vi "External EEPROM.vi"(8 "error in":errorcluster) -> (0 "error out":errorcluster, 2 "Pass?":bool, 3 "VISA resource name out":refnum<visa-resource-name>)   [LabVIEW 2009]
uses:
  Digit IO PCI 6503/Digit IO control.ctl
  Global/Global 1.vi
  <vilib>/Instr/_visa.llb/VISA Configure Serial Port (Instr).vi
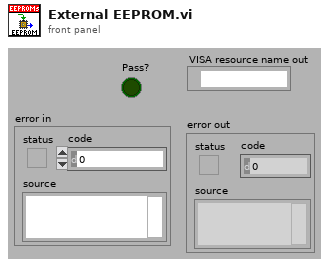
[diagram p1: front panel]
types:
  T1 = typedef "Digit IO control.ctl" = enum16{"Pull X1_4 Low", "Disconnect Pull X1_4 Low", "Down Cylinder", "Disconnect Down Cylinder", "Load X1_1_5", "Disconnect Load X1_1_5", "Measu X1_1_5", "Disconnect Measu X1_1_5", "Measu Z1_1_5", "Disconnect Measu Z1_1_5", "Power X1_1", "Disconnect Power X1_1", "RS232 Power", "Disconnect RS232 Power", "Card Cylinder", "Disconnect Card Cylinder", "Fail LED", "Disconnect Fail LED", "LCA Power", "Disconnect LCA Power", "BeyondCylinderDowndigit", "Disconnect BeyondCylinderDowendigit", "Frequency", "Disconnect Frequency", "Measu Current", "Disconnect Measu Current", "Measu current_1", "Disconnect Measu current_1", "Digit ALL", "Disconnect Digit ALL", "PASS LED", "Disconnect PASS LED", "Load Z1_1_3", "Disconnect Load Z1_1_3", "RS232 Connect", "Disconnect RS232 Connect", "Power Z1_7", "Disconnect Power Z1_7", "Pull Z_1_5  low", "Disconnect Pull Z_1_5  low", "Connect LCA_1", "Disconnect LCA_1", "short LCA", "Disconnect short LCA", "PT100", "Disconnect PT100", "NO connect", "Disconnect NO connect"}
  T2 = cluster{"People":string, "product  number":string, "Test time":string, "VHeatFuse_noload":string, "VHeatFuse_load":string, "VoverrideDiode":string, "Test firmware upload via X1":string, "TemperAddress":string, "Troom":string, "TLCU":string, "Adjustment factor":string, "MeasuredFreq":string, "I2C communication":string, "Light-emitting diode on Z2":string, "Battery warning/inhibit":string, "Reset by IC10":string, "External EEPROM":string, "RFID card detection and reading RFID":string, "Production parameters in internal EEPROM":string, "Current consumption in sleep mode":string, "Application and database upload":string, "Test result":string, "Table head[22]":string, "Table head[23]":string}
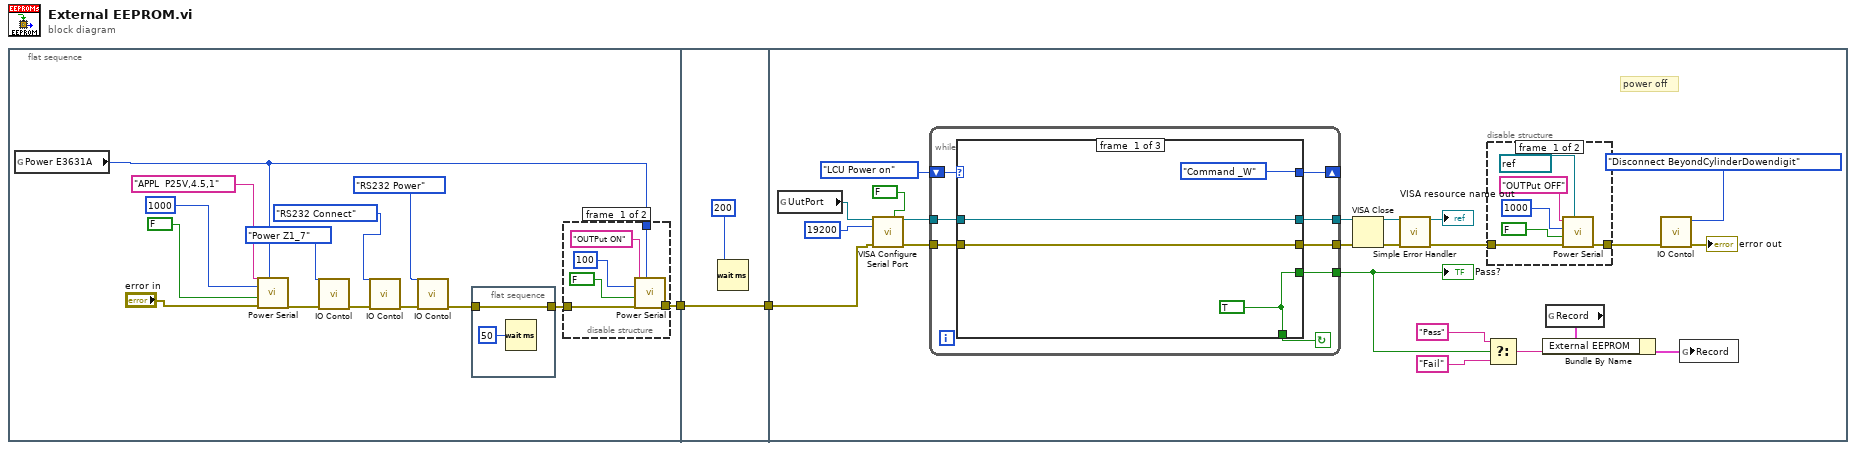
[diagram p0: block diagram]
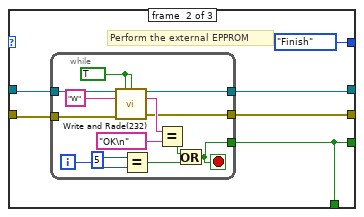
[diagram p4: hidden frame]
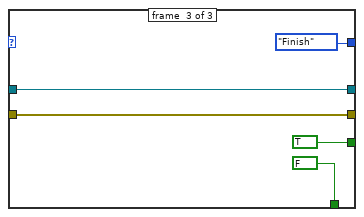
[diagram p5: hidden frame]
diagram:
  n1 = flat-sequence {
    tunnel: [w4] -> w1
    tunnel: [w26] -> w2
    tunnel: w1 -> [w26]
    tunnel: w2 -> [w35]
    frame #0 {
      n2 = global read "Global 1.vi" "Power E3631A"() -> (w7:i32)
      n3 = call "Power Serial.vi"("VISA Resource Address"=w7, "error in (no error)"="error in", "Rd?"=FALSE, "Delay"=1000, "IN"="APPL  P25V,4.5,1" ("In")) -> ("error out"=w11:errorcluster)  [unwired: 6 out]
      n4 = call "IO Contol.vi"("error in"=w11, "IO Operation"=Digit_IO_control."Power Z1_7" ("Enum")) -> ("error out"=w12:errorcluster)  [unwired: 9 out]
      n5 = call "IO Contol.vi"("error in"=w12, "IO Operation"=Digit_IO_control."RS232 Connect" ("Enum")) -> ("error out"=w13:errorcluster)  [unwired: 9 out]
      n6 = call "IO Contol.vi"("error in"=w13, "IO Operation"=Digit_IO_control."RS232 Power" ("Enum")) -> ("error out"=w6:errorcluster)  [unwired: 9 out]
      n7 = flat-sequence {
        tunnel: [w25] -> w5
        tunnel: w6 -> [w25]
        frame #0 {
          n8 = Wait (ms)(milliseconds to wait=u32 50) -> ()  [unwired: 1 out]
        }
      }
      n9 = disable-structure shown="Enabled" {
        disable-tunnel: w7 -> [w19 _]
        disable-tunnel: w5 -> [w18 w23]
        disable-tunnel: [w17 w23] -> w4
        frame #0 {
          n10 = call "Power Serial.vi"("VISA Resource Address"=w19, "error in (no error)"=w18, "Rd?"=FALSE, "Delay"=100, "IN"="OUTPut ON" ("In")) -> ("error out"=w17:errorcluster)  [unwired: 5 in, 1 out]
        }
        frame #1 {
        }
      }
    }
    frame #1 {
      n11 = Wait (ms)(milliseconds to wait=u32 200) -> ()  [unwired: 1 out]
    }
    frame #2 {
      # "power off"
      n12 = global read "Global 1.vi" "UutPort"() -> (w34:refnum<visa-resource-name>)
      n13 = call-poly "VISA Configure Serial Port"("VISA resource name"=w34, "Enable Termination\nChar (T)"=FALSE ("Enable Termination\nChar (T)"), "baud rate (9600)"=u32 19200, "error in (no error)"=w35) -> ("VISA resource name out"=w38:refnum<visa-resource-name>, "error out"=w36:errorcluster)  [unwired: 3 in, 7 out]
      n14 = while {
        shift-right: [w55] -> _
        shift-left: enum16{"LCU Power on", "Command _W", "Finish"}."LCU Power on" -> [w56]
        tunnel: [w61] -> w39
        tunnel: w38 -> [w60]
        tunnel: [w59] -> w37
        tunnel: w36 -> [w58]
        tunnel: [w57] -> w30
        stop <- w62 continue-if-true
        n15 = case shown="\"Command _W\"" w56 {
          tunnel: [enum16{"LCU Power on", "Command _W", "Finish"}."Command _W" enum16{"LCU Power on", "Command _W", "Finish"}."Finish" enum16{"LCU Power on", "Command _W", "Finish"}."Finish"] -> w55
          tunnel: [w65 w67 FALSE] -> w62
          tunnel: [w66 w69 w88] -> w61
          tunnel: w60 -> [w66 w72 w88]
          tunnel: [w63 w70 w86] -> w59
          tunnel: w58 -> [w63 w71 w86]
          tunnel: [w65 w67 TRUE] -> w57
          frame #0 {
            w65 = TRUE
          }
          frame #1 {
            # "Perform the external EPPROM"
            n16 = while {
              tunnel: w72 -> [w85]
              tunnel: w71 -> [w84]
              tunnel: [w79] -> w70
              tunnel: [w78] -> w69
              tunnel: [w73] -> w67
              i -> [w75]
              stop <- w73 stop-if-true
              w83 = TRUE ("write")
              n17 = call "Write and Rade(232).vi"("VISA resource name in"=w85, "write"=w83, "read"=w83, "string to write"="W", "error in"=w84) -> ("VISA resource name out"=w78:refnum<visa-resource-name>, "read string"=w81:string, "error out"=w79:errorcluster)  [unwired: 3 in, 5 out]
              n18 = Equal?(x=5, y=w75) -> (x = y?=w74:bool)
              n19 = Equal?(x=w81, y="OK\n") -> (x = y?=w77:bool)
              n20 = Or(x=w77, y=w74) -> (x .or. y?=w73:bool)
            }
          }
          frame #2 {
          }
        }
      }
      "VISA resource name out" <- w39
      "Pass?" <- w30
      n21 = VISA Close(VISA resource name=w39, error in (no error)=w37) -> (error out=w41:errorcluster)
      n22 = call <vilib>:"Simple Error Handler.vi"("error in (no error)"=w41) -> ("error out"=w45:errorcluster)  [unwired: 1 in, 7 out]
      n23 = disable-structure shown="Enabled" {
        disable-tunnel: [w50 w54] -> w46
        disable-tunnel: w45 -> [w48 w54]
        frame #0 {
          n24 = call "Power Serial.vi"("VISA Resource Address"=refnum<visa-resource-name> "COM1", "error in (no error)"=w48, "Rd?"=FALSE, "Delay"=1000, "IN"="OUTPut OFF" ("In")) -> ("error out"=w50:errorcluster)  [unwired: 5 in, 1 out]
        }
        frame #1 {
        }
      }
      n25 = Select(t="Pass", s=w30, f="Fail") -> (s? t:f=w29:string)
      n26 = global read "Global 1.vi" "Record"() -> (w33:T2)
      n27 = Bundle By Name(cluster=w33, "External EEPROM"=w29) -> (w28:T2)
      n28 = call "IO Contol.vi"("error in"=w46, "IO Operation"=Digit_IO_control."Disconnect BeyondCylinderDowendigit" ("Enum")) -> ("error out"=→"error out":errorcluster)  [unwired: 9 out]
      n29 = global write "Global 1.vi" "Record"(w28) -> ()
    }
  }
